vi "Helper - Image To UTM.vi"(2 "Image Descriptor":T3={"Upper-Left Corner Coordinates"={"UTM Zone"=0.0, "Hemisphere"=enum."North", "East"=0.0, "North"=0.0}, "Meters/Pixel"=42.294203} {"Upper-Left Corner Coordinates"."North" format="%#_10f"; "Upper-Left Corner Coordinates"."East" format="%#_8f"}, 4 "Pixel Coordinates":cluster{"X":i32, "Y":i32}) -> (0 "Waypoint":T1 {"UTM Location"."North" format="%#_10f"; "UTM Location"."East" format="%#_8f"}, 1 "UTM Location":T2 {"North" format="%#_10f"; "East" format="%#_8f"})   [LabVIEW 2011]
doc: "Converts image pixels to UTM coordinates using an Image Descriptor.\n-Jason"
uses:
  0-OCU/0 Code/mission input/0-Image Descriptor.ctl
  2 Typedefs/UTM Location.ctl
  0x2-OCU-Think Comm/0x2 Typedefs/ocuWaypoint.ctl
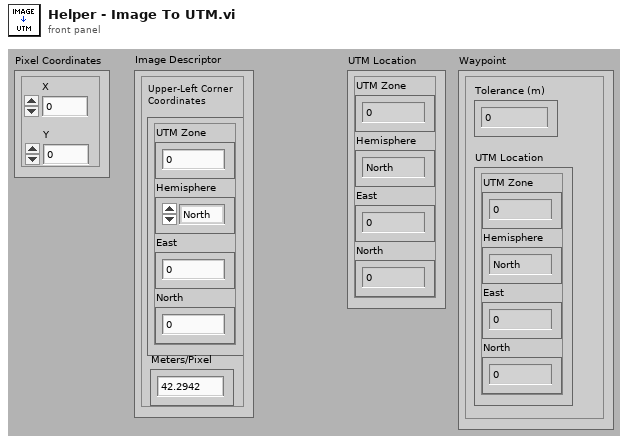
[diagram p1: front panel]
types:
  T1 = typedef "ocuWaypoint.ctl" = cluster{"Tolerance (m)":dbl, "UTM Location":T2}
  T2 = typedef "UTM Location.ctl" = cluster{"UTM Zone":dbl, "Hemisphere":enum16{"North", "South"}, "East":dbl, "North":dbl}
  T3 = typedef "0-Image Descriptor.ctl" = cluster{"Upper-Left Corner Coordinates":T2, "Meters/Pixel":dbl}
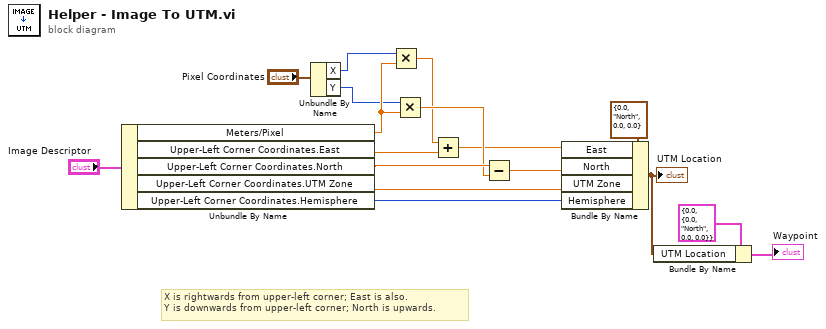
[diagram p0: block diagram]
diagram:
  # "X is rightwards from upper-left corner; East is also.\nY is downwards from upper-left corner; North is upwards."
  n1 = Unbundle By Name("Image Descriptor") -> ("Meters/Pixel"=w13:dbl, "Upper-Left Corner Coordinates.East"=w12:dbl, "Upper-Left Corner Coordinates.North"=w11:dbl, "Upper-Left Corner Coordinates.UTM Zone"=w15:dbl, "Upper-Left Corner Coordinates.Hemisphere"=w14:enum16{"North", "South"})
  n2 = Unbundle By Name("Pixel Coordinates") -> ("X"=w3:i32, "Y"=w2:i32)
  n3 = Multiply(x=w3, y=w13) -> (x*y=w9:dbl)
  n4 = Multiply(x=w2, y=w13) -> (x*y=w10:dbl)
  n5 = Add(x=w9, y=w12) -> (x+y=w8:dbl)
  n6 = Subtract(x=w11, y=w10) -> (x-y=w7:dbl)
  n7 = Bundle By Name(cluster=T2 {"UTM Zone"=0.0, "Hemisphere"=enum."North", "East"=0.0, "North"=0.0} ("UTM Location 2"), "East"=w8, "North"=w7, "UTM Zone"=w15, "Hemisphere"=w14) -> (w4:T2)
  "UTM Location" <- w4
  n8 = Bundle By Name(cluster=T1 {"Tolerance (m)"=0.0, "UTM Location"={"UTM Zone"=0.0, "Hemisphere"=enum."North", "East"=0.0, "North"=0.0}} ("Waypoint 2"), "UTM Location"=w4) -> (→"Waypoint":T1)
